vi "1. ControlRealTimeEx1.vi"() -> ()   [LabVIEW 2011]
panel:
  in  "Value":dbl
  out "GetDataPCounter":string[][](array[string])
  in  "HVAC System IP Address":string(combo)="130.237.50.30"
  out "Real-time CO2 data comming from mote with id 1":dbl(graph)
  in  "Password":string
  in  "Username":string
  out "Access to HVAC Msg":errorcluster={"status"=FALSE, "code"=0, "source"="Please Wait ..."}
  out "Actuation Result Msg":string
  out "GetDataPlcs Output 4":string[][](array[string])
  out "GetDataPlcs Output 3":string[][](array[string])
  out "GetDataPlcs Output 2":string[][](array[string])
  out "GetDataPlcs Output 1":string[][](array[string])
  out "GetDataMotes Output 6":string[][](array[string])
  out "GetDataMotes Output 5":string[][](array[string])
  out "GetDataMotes Output 4":string[][](array[string])
  out "GetDataMotes Output 3":string[][](array[string])
  out "GetDataMotes Output 2":string[][](array[string])
  out "GetDataMotes Output 1":string[][](array[string])
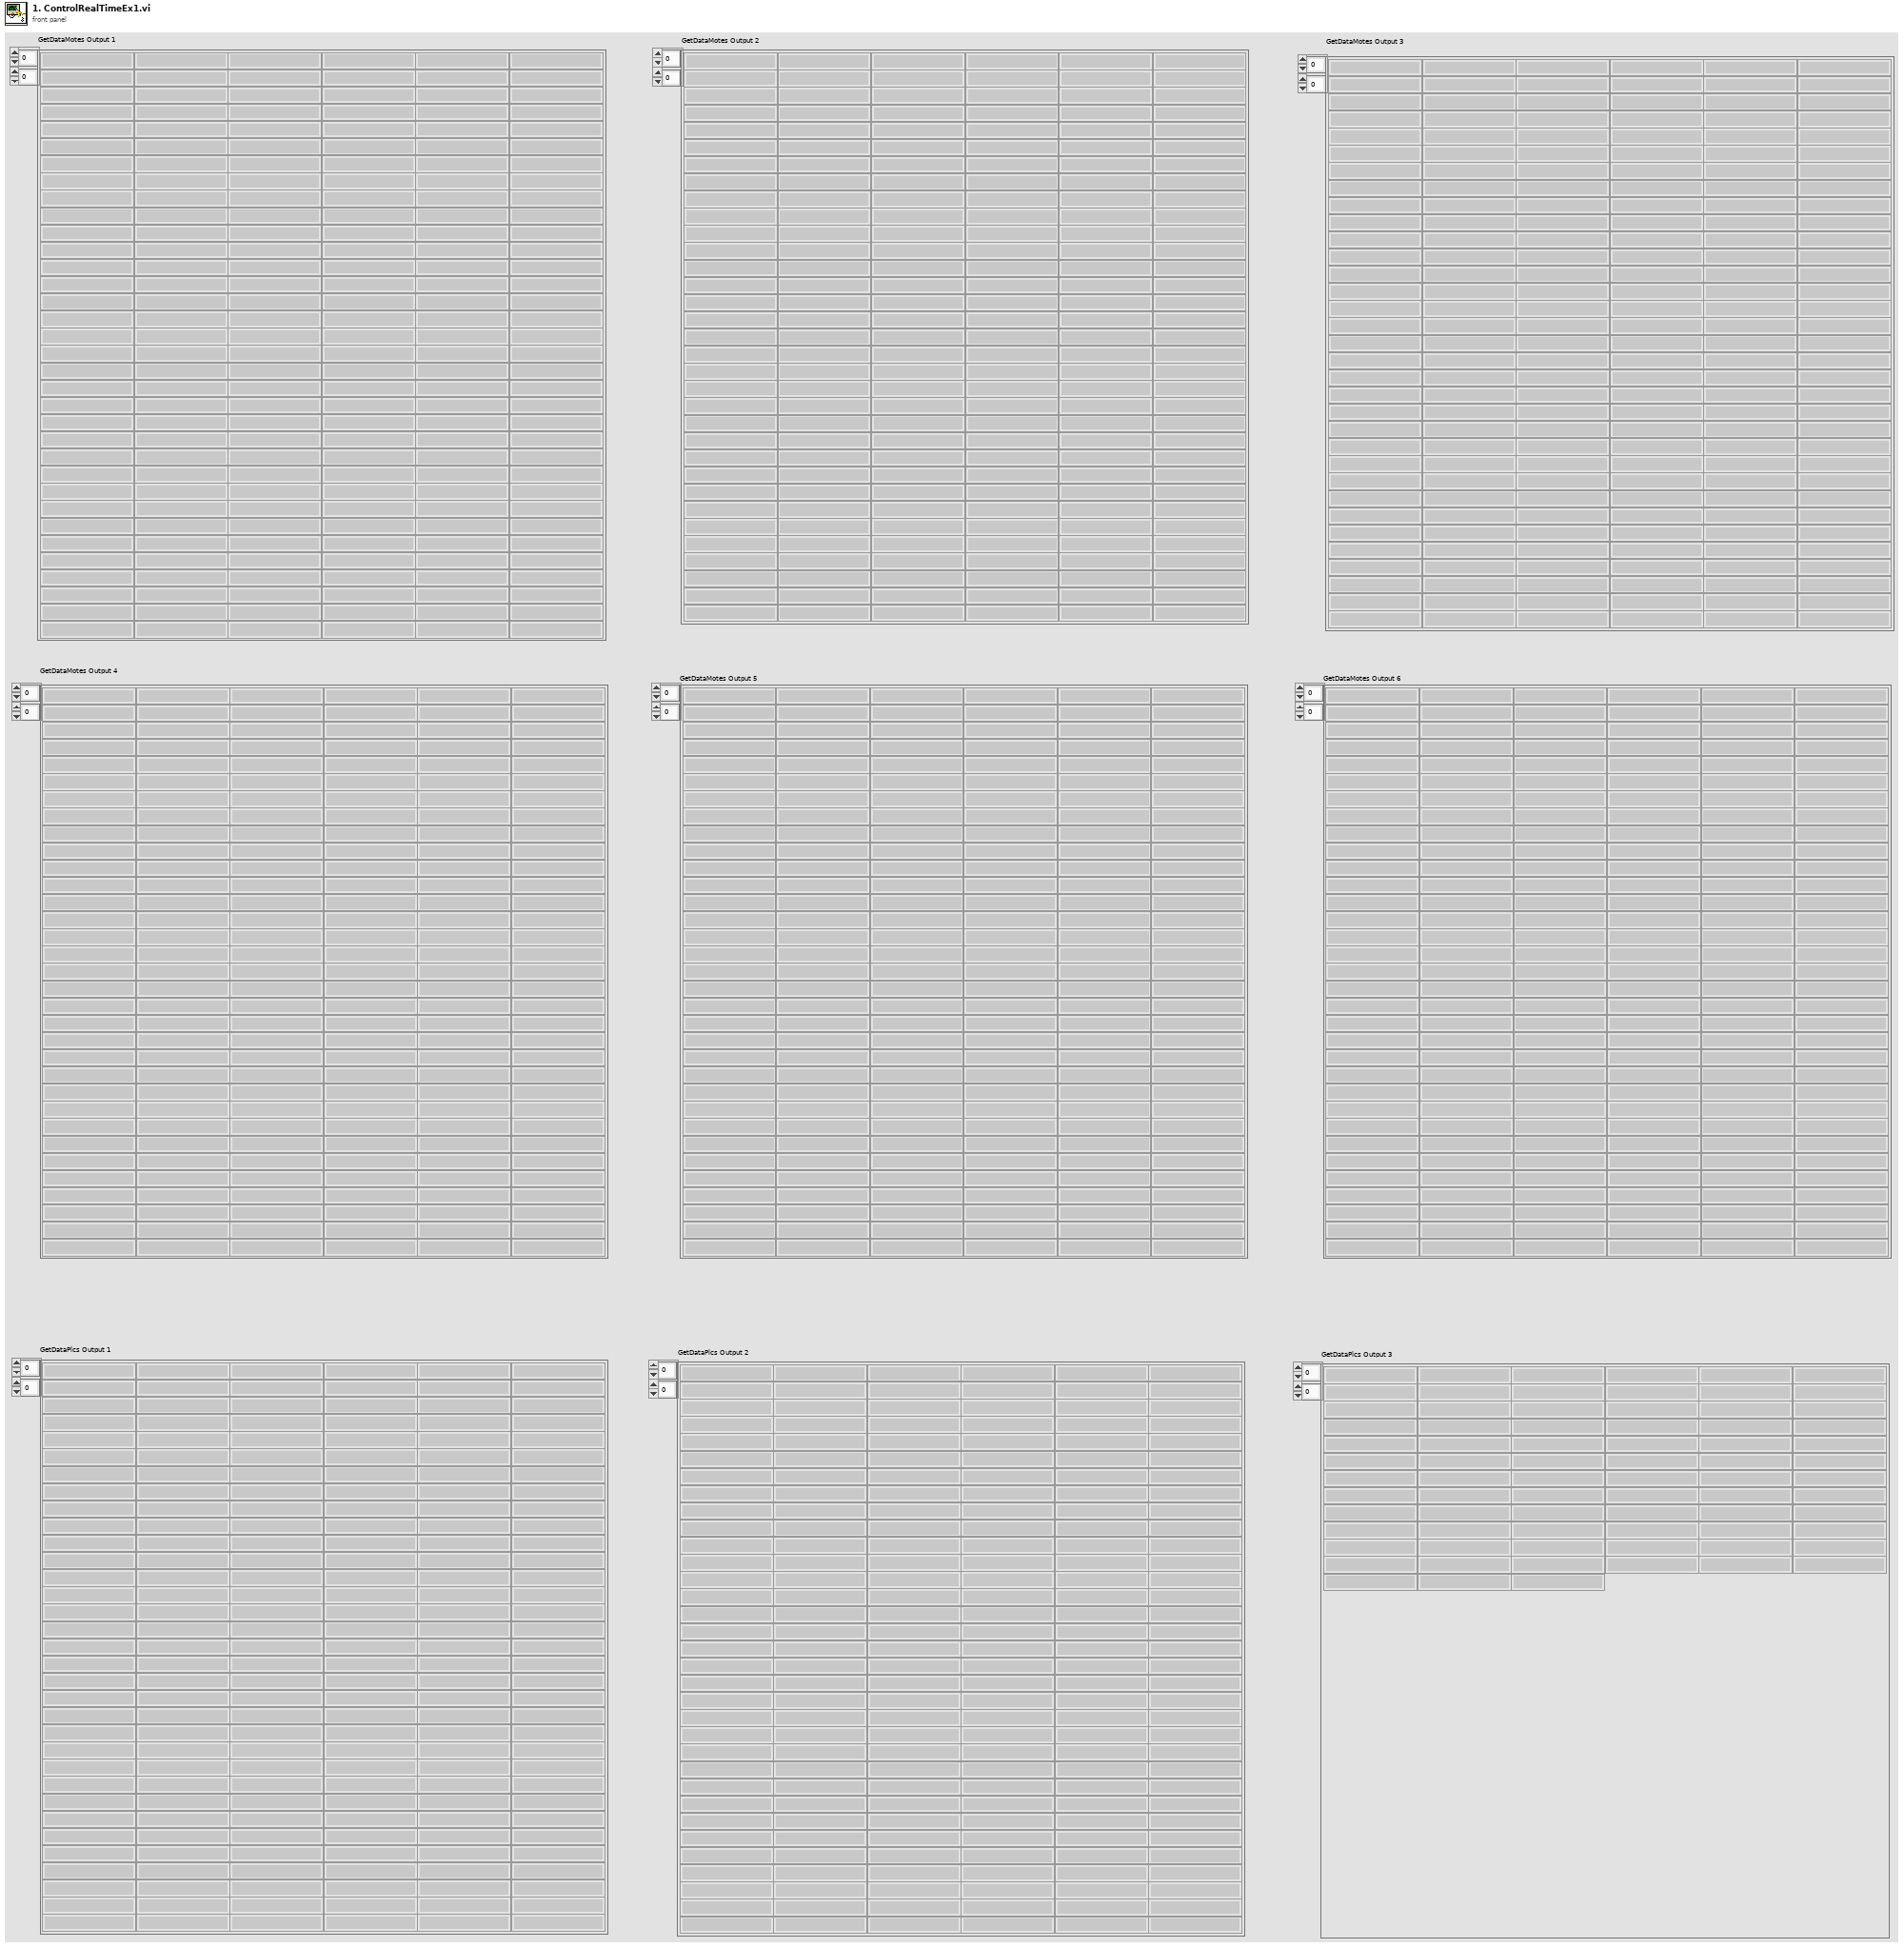
[diagram p1: front panel]
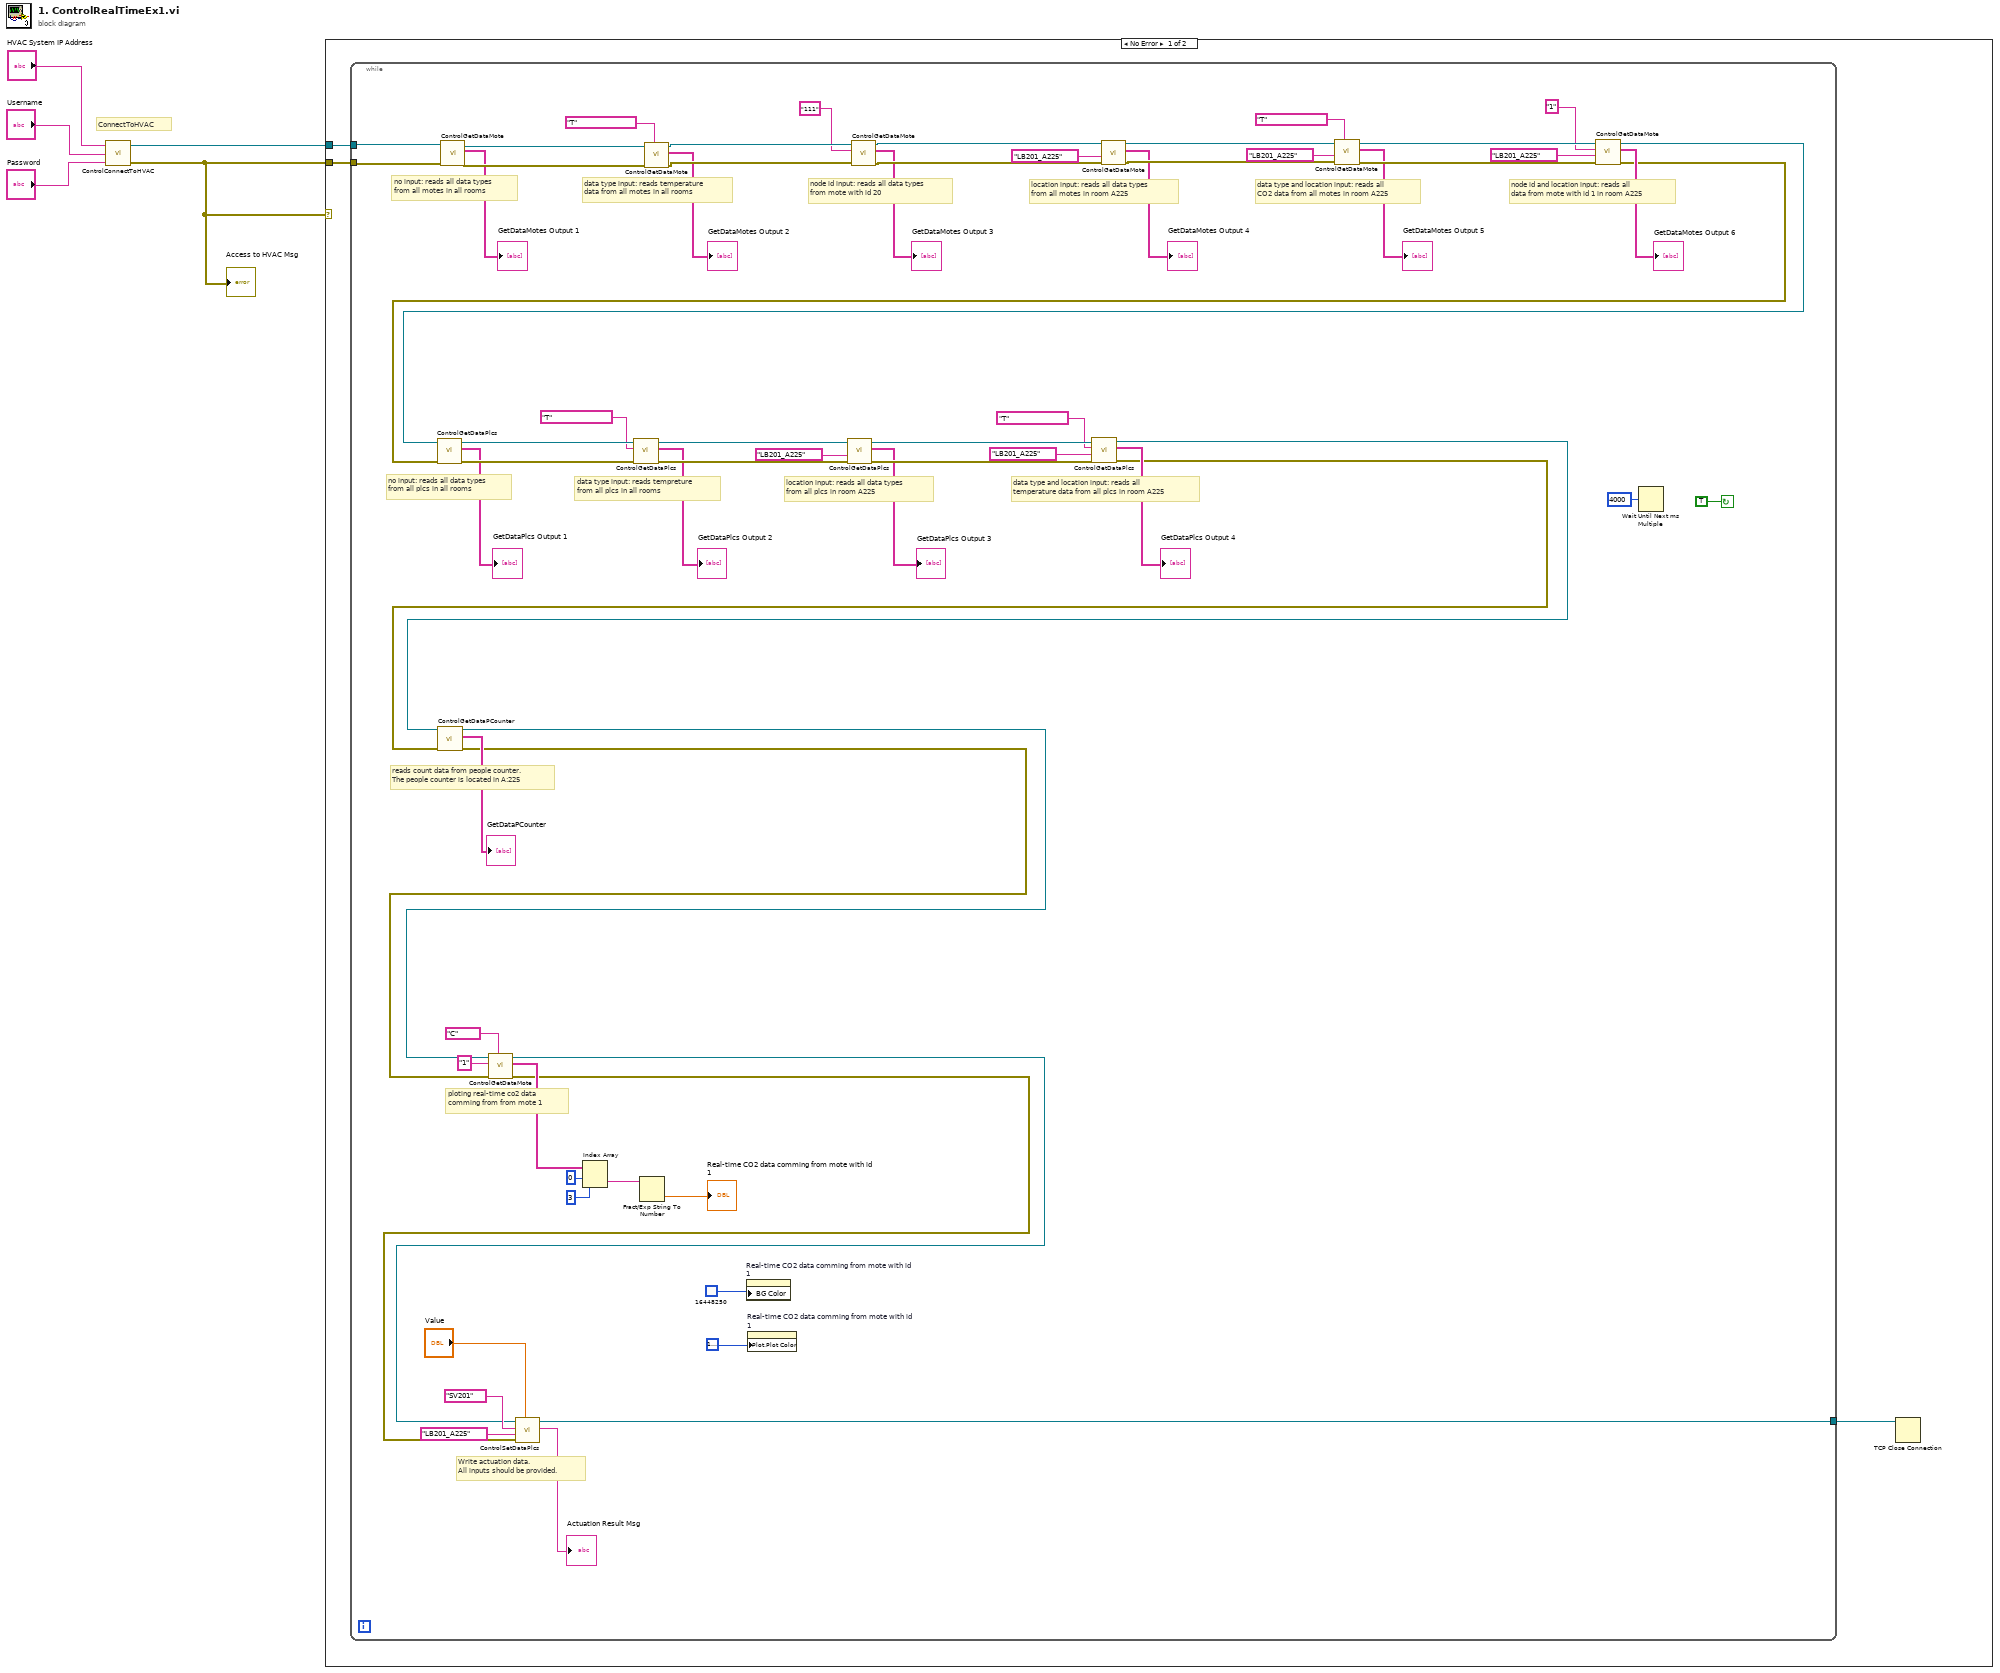
[diagram p0: block diagram]
diagram:
  # "ConnectToHVAC"
  n1 = call "ControlConnectToHVAC.vi"("Password"="Password", "Username"="Username", "IP Address"="HVAC System IP Address") -> ("error out"=w4:errorcluster, "connection ID out"=w5:refnum<k5>)  [unwired: 1 in]
  "Access to HVAC Msg" <- w4
  n2 = case shown="No Error" w4 {
    tunnel: w5 -> [w8 _]
    tunnel: w4 -> [w7 _]
    frame No Error {
      n3 = while {
        tunnel: w8 -> [w69]
        tunnel: w7 -> [w70]
        tunnel: [w12] -> w6
        stop <- TRUE continue-if-true
        # "Write actuation data. \nAll inputs should be provided."
        # "reads count data from people counter.\nThe people counter is located in A:225"
        # "ploting real-time co2 data \ncomming from from mote 1"
        # "data type and location input: reads all \ntemperature data from all plcs in room A225"
        # "location input: reads all data types \nfrom all plcs in room A225"
        # "data type input: reads tempreture \nfrom all plcs in all rooms"
        # "no input: reads all data types \nfrom all plcs in all rooms"
        # "node id and location input: reads all \ndata from mote with id 1 in room A225"
        # "data type and location input: reads all \nCO2 data from all motes in room A225"
        # "location input: reads all data types \nfrom all motes in room A225"
        # "node id input: reads all data types\nfrom mote with id 20"
        # "data type input: reads temperature \ndata from all motes in all rooms"
        # "no input: reads all data types \nfrom all motes in all rooms"
        n4 = call "ControlGetDataMote.vi"("error in"=w70, "connection ID in"=w69) -> ("error out"=w59:errorcluster, "output array"=→"GetDataMotes Output 1":string[][], "connection ID out"=w60:refnum<k5>)  [unwired: 7 in]
        n5 = call "ControlGetDataMote.vi"("Data Type"="T", "error in"=w59, "connection ID in"=w60) -> ("error out"=w68:errorcluster, "output array"=→"GetDataMotes Output 2":string[][], "connection ID out"=w67:refnum<k5>)  [unwired: 6 in]
        n6 = property on="Real-time CO2 data comming from mote with id 1" class="WFChart (strict)"("BG Color"=u32 16448250) -> ()  [unwired: 2 in, 2 out]
        n7 = property on="Real-time CO2 data comming from mote with id 1" class="WFChart (strict)"("Plot.Plot Color"=u32 16777222) -> ()  [unwired: 2 in, 2 out]
        n8 = call "ControlGetDataMote.vi"("error in"=w68, "Node ID"="111", "connection ID in"=w67) -> ("error out"=w65:errorcluster, "output array"=→"GetDataMotes Output 3":string[][], "connection ID out"=w66:refnum<k5>)  [unwired: 6 in]
        n9 = call "ControlGetDataMote.vi"("error in"=w65, "Location"="LB201_A225", "connection ID in"=w66) -> ("error out"=w63:errorcluster, "output array"=→"GetDataMotes Output 4":string[][], "connection ID out"=w64:refnum<k5>)  [unwired: 6 in]
        n10 = call "ControlGetDataMote.vi"("Data Type"="T", "error in"=w63, "Location"="LB201_A225", "connection ID in"=w64) -> ("error out"=w61:errorcluster, "output array"=→"GetDataMotes Output 5":string[][], "connection ID out"=w62:refnum<k5>)  [unwired: 5 in]
        n11 = call "ControlGetDataMote.vi"("error in"=w61, "Location"="LB201_A225", "Node ID"="1", "connection ID in"=w62) -> ("error out"=w38:errorcluster, "output array"=→"GetDataMotes Output 6":string[][], "connection ID out"=w40:refnum<k5>)  [unwired: 5 in]
        n12 = call "ControlGetDataPlcs.vi"("error in"=w38, "connection ID in"=w40) -> ("error out"=w49:errorcluster, "output array"=→"GetDataPlcs Output 1":string[][], "connection ID out"=w50:refnum<k5>)  [unwired: 6 in]
        n13 = call "ControlGetDataPlcs.vi"("error in"=w49, "Data Type"="T", "connection ID in"=w50) -> ("error out"=w48:errorcluster, "output array"=→"GetDataPlcs Output 2":string[][], "connection ID out"=w47:refnum<k5>)  [unwired: 5 in]
        n14 = call "ControlGetDataPlcs.vi"("error in"=w48, "Location"="LB201_A225", "connection ID in"=w47) -> ("error out"=w45:errorcluster, "output array"=→"GetDataPlcs Output 3":string[][], "connection ID out"=w46:refnum<k5>)  [unwired: 5 in]
        n15 = call "ControlGetDataPlcs.vi"("error in"=w45, "Location"="LB201_A225", "Data Type"="T", "connection ID in"=w46) -> ("error out"=w10:errorcluster, "output array"=→"GetDataPlcs Output 4":string[][], "connection ID out"=w9:refnum<k5>)  [unwired: 4 in]
        n16 = call "ControlGetDataPCounter.vi"("error in"=w10, "connection ID in"=w9) -> ("error out"=w20:errorcluster, "output array"=→"GetDataPCounter":string[][], "connection ID out"=w21:refnum<k5>)  [unwired: 7 in]
        n17 = call "ControlGetDataMote.vi"("Data Type"="C", "error in"=w20, "Node ID"="1", "connection ID in"=w21) -> ("error out"=w24:errorcluster, "output array"=w29:string[][], "connection ID out"=w25:refnum<k5>)  [unwired: 5 in]
        n18 = call "ControlSetDataPlcs.vi"("data"="Value", "error in"=w24, "Location"="LB201_A225", "Node ID"="SV201", "connection ID in"=w25) -> ("Output Msg"=→"Actuation Result Msg":string, "connection ID out"=w12:refnum<k5>)  [unwired: 3 in, 1 out]
        n19 = Index Array(array=w29, index (row)=0, index (col)=3 ("disabled index (col)")) -> (element=w26:string)
        n20 = Fract/Exp String To Number(string=w26) -> (number=→"Real-time CO2 data comming from mote with id 1":dbl)  [unwired: 3 in, 1 out]
        n21 = Wait Until Next ms Multiple(millisecond multiple=u32 4000) -> ()  [unwired: 1 out]
      }
      n22 = TCP Close Connection(connection ID=w6) -> ()  [unwired: 2 in, 2 out]
    }
    frame Error {
    }
  }
